vi "add Character in two side of string.vi"(7 "Add Character":string="\"", 11 "Sting In":string) -> (3 "String Out":string)   [LabVIEW 2021, in "DataBase_SQL.lvclass"]
uses:
  <userlib>/John_Lib/DataBase/DataBase_SQL/DataBase_SQL.lvclass
  <userlib>/John_Lib/DataBase/DataBase_SQL/DataBase_SQL.lvclass/DataBase_SQL.ctl
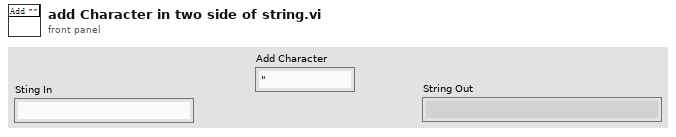
[diagram p1: front panel]
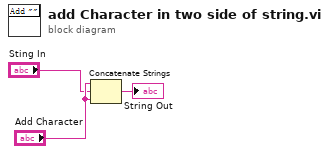
[diagram p0: block diagram]
diagram:
  n1 = Concatenate Strings("Add Character", "Sting In", "Add Character") -> (→"String Out":string)
